vi "DAQClose.vi"(8 "error in":errorcluster, 9 "Functions":T3(ring)=enum."Measurement", 10 "Tasks In":T1, 11 "DAQ Channels":T2) -> (0 "error out":errorcluster)   [LabVIEW 2015]
uses:
  <vilib>/DAQmx/write.llb/DAQmx Write (Analog 1D DBL NChan 1Samp).vi
  <vilib>/DAQmx/create/channels.llb/DAQmx Create Channel (AO-Voltage-Basic).vi
  <vilib>/DAQmx/miscellaneous.llb/DAQmx Fill In Error Info.vi
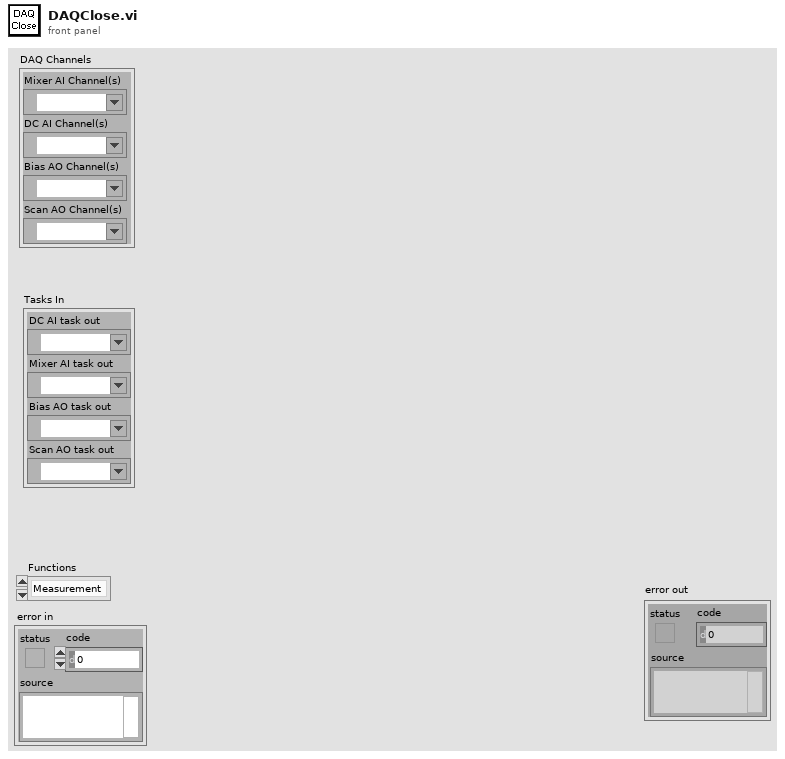
[diagram p1: front panel]
types:
  T1 = cluster{"DC AI task out":refnum<k21>, "Mixer AI task out":refnum<k21>, "Bias AO task out":refnum<k21>, "Scan AO task out":refnum<k21>}
  T2 = cluster{"Mixer AI Channel(s)":tag, "DC AI Channel(s)":tag, "Bias AO Channel(s) ":tag, "Scan AO Channel(s)":tag}
  T3 = enum32{"Calibration", "Fast Scan", "Measurement"}
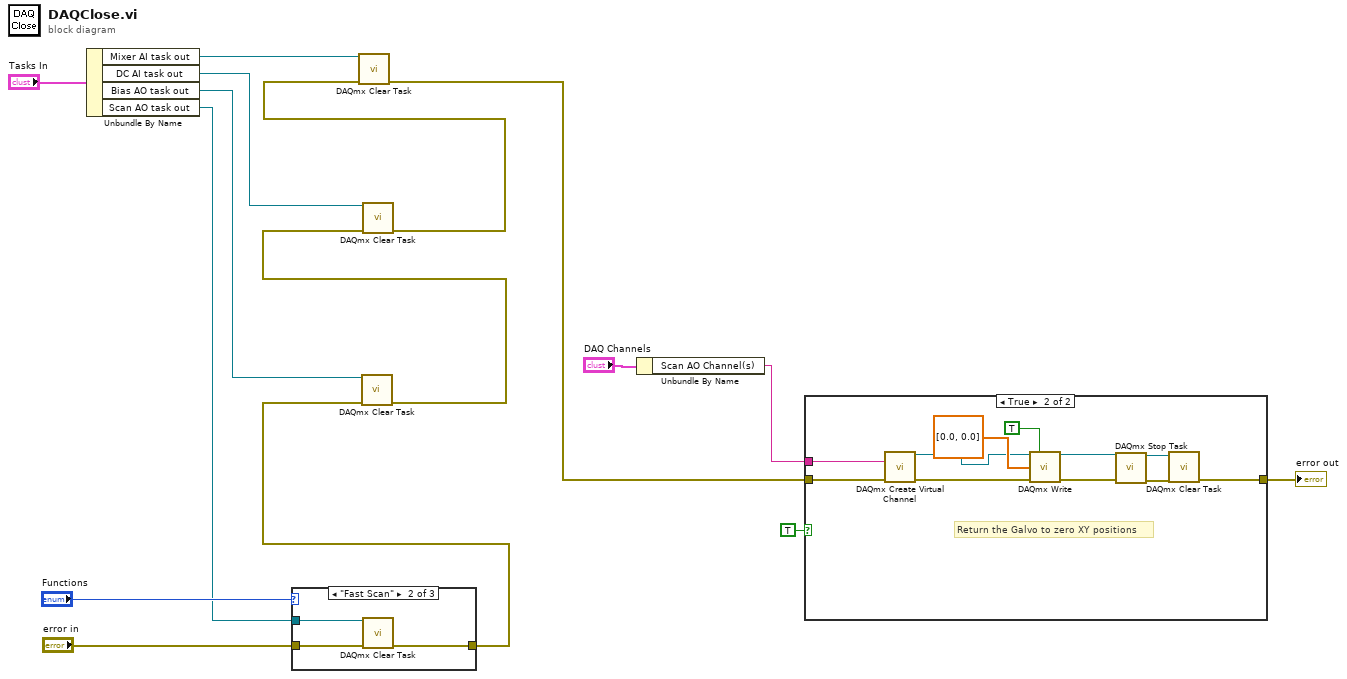
[diagram p0: block diagram]
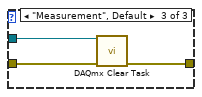
[diagram p4: hidden frame]
diagram:
  n1 = Unbundle By Name("Tasks In") -> ("Mixer AI task out"=w4:refnum<k21>, "DC AI task out"=w9:refnum<k21>, "Bias AO task out"=w10:refnum<k21>, "Scan AO task out"=w14:refnum<k21>)
  n2 = case shown="\"Fast Scan\"" "Functions" {
    tunnel: w14 -> [_ w17 w22]
    tunnel: "error in" -> [w16 w19 w21]
    tunnel: [w16 w18 w20] -> w12
    frame "Calibration" {
    }
    frame "Fast Scan" {
      n3 = call <vilib>:"DAQmx Clear Task.vi"("task in"=w17, "error in"=w19) -> ("error out"=w18:errorcluster)  [unwired: 13 in]
    }
    frame "Measurement", Default {
      n4 = call <vilib>:"DAQmx Clear Task.vi"("task in"=w22, "error in"=w21) -> ("error out"=w20:errorcluster)  [unwired: 13 in]
    }
  }
  n5 = call <vilib>:"DAQmx Clear Task.vi"("task in"=w10, "error in"=w12) -> ("error out"=w11:errorcluster)  [unwired: 13 in]
  n6 = call <vilib>:"DAQmx Clear Task.vi"("task in"=w9, "error in"=w11) -> ("error out"=w3:errorcluster)  [unwired: 13 in]
  n7 = call <vilib>:"DAQmx Clear Task.vi"("task in"=w4, "error in"=w3) -> ("error out"=w2:errorcluster)  [unwired: 13 in]
  n8 = Unbundle By Name("DAQ Channels") -> ("Scan AO Channel(s)"=w6:tag)
  n9 = case shown="True" TRUE {
    tunnel: [w23 w24] -> w7
    tunnel: w6 -> [_ w32]
    tunnel: w2 -> [w23 w29]
    frame False {
    }
    frame True {
      # "Return the Galvo to zero XY positions"
      n10 = call-poly <vilib>:"DAQmx Create Virtual Channel.vi"("physical channels"=w32, "error in"=w29) -> ("task out"=w31:refnum<k21>, "error out"=w30:errorcluster)  [unwired: 12 in]
      n11 = call-poly <vilib>:"DAQmx Write.vi"("task/channels in"=w31, "auto start"=TRUE, "data"=dbl[] [0.0, 0.0], "error in"=w30) -> ("task out"=w27:refnum<k21>, "error out"=w28:errorcluster)  [unwired: 9 in, 1 out]
      n12 = call <vilib>:"DAQmx Stop Task.vi"("task/channels in"=w27, "error in"=w28) -> ("task out"=w26:refnum<k21>, "error out"=w25:errorcluster)  [unwired: 12 in]
      n13 = call <vilib>:"DAQmx Clear Task.vi"("task in"=w26, "error in"=w25) -> ("error out"=w24:errorcluster)  [unwired: 13 in]
    }
  }
  "error out" <- w7
